vi "Read Control Voltage.vi"(8 "error in":errorcluster, 11 "task in":refnum<k21>) -> (0 "error out":errorcluster, 2 "Current Control Voltage":dbl format="%0.2f", 3 "task out":refnum<k21>)   [LabVIEW 2009, in "Varian.lvlib"]
doc: "Reads the current control voltage from the DAQ."
uses:
  Varian.lvlib
  <vilib>/DAQmx/read.llb/DAQmx Read (Analog DBL 1Chan 1Samp).vi
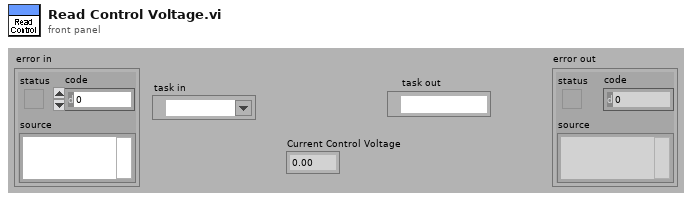
[diagram p1: front panel]
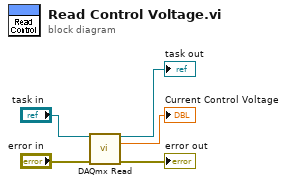
[diagram p0: block diagram]
diagram:
  n1 = call-poly <vilib>:"DAQmx Read.vi"("task/channels in"="task in", "error in"="error in") -> ("task out"=→"task out":refnum<k21>, "data"=→"Current Control Voltage":dbl, "error out"=→"error out":errorcluster)  [unwired: 11 in]
